vi "curve_fitter.vi"(8 "Path 4":path, 9 "Path 3":path, 10 "Path 2":path, 11 "Path":path) -> (0 "interleaved array":dbl[](array[numeric]), 1 "RMS":dbl, 2 "Standard Dev":dbl, 3 "Arithmetic Mean":dbl)   [LabVIEW 2019]
uses:
  <vilib>/Analysis/6fits.llb/Curve Fitting Criteria.ctl
  <vilib>/Utility/file.llb/Read Delimited Spreadsheet (string).vi
  <vilib>/Analysis/NI_AALPro.lvlib
panel:
  out "Total Samples":dbl
  out "Variance":dbl
  out "Array":dbl[][](array[numeric])
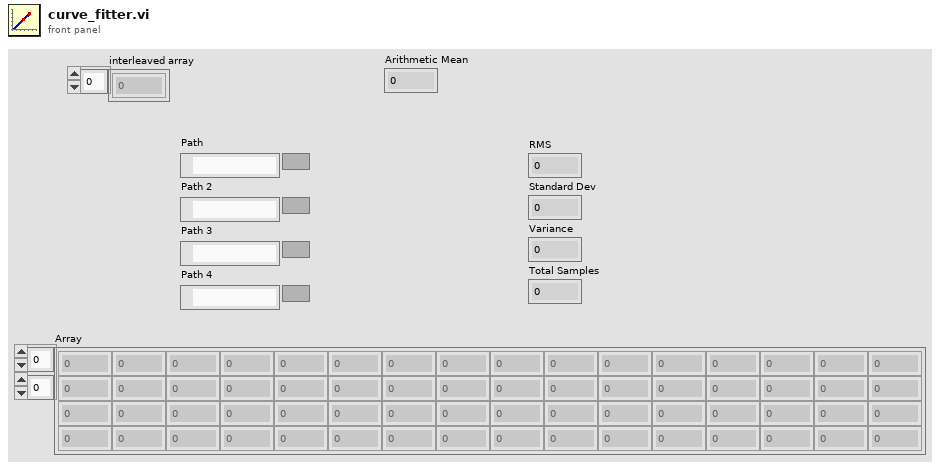
[diagram p1: front panel]
types:
  T1 = typedef "NI_AALPro.lvlib/Curve Fitting Criteria.ctl" = u16
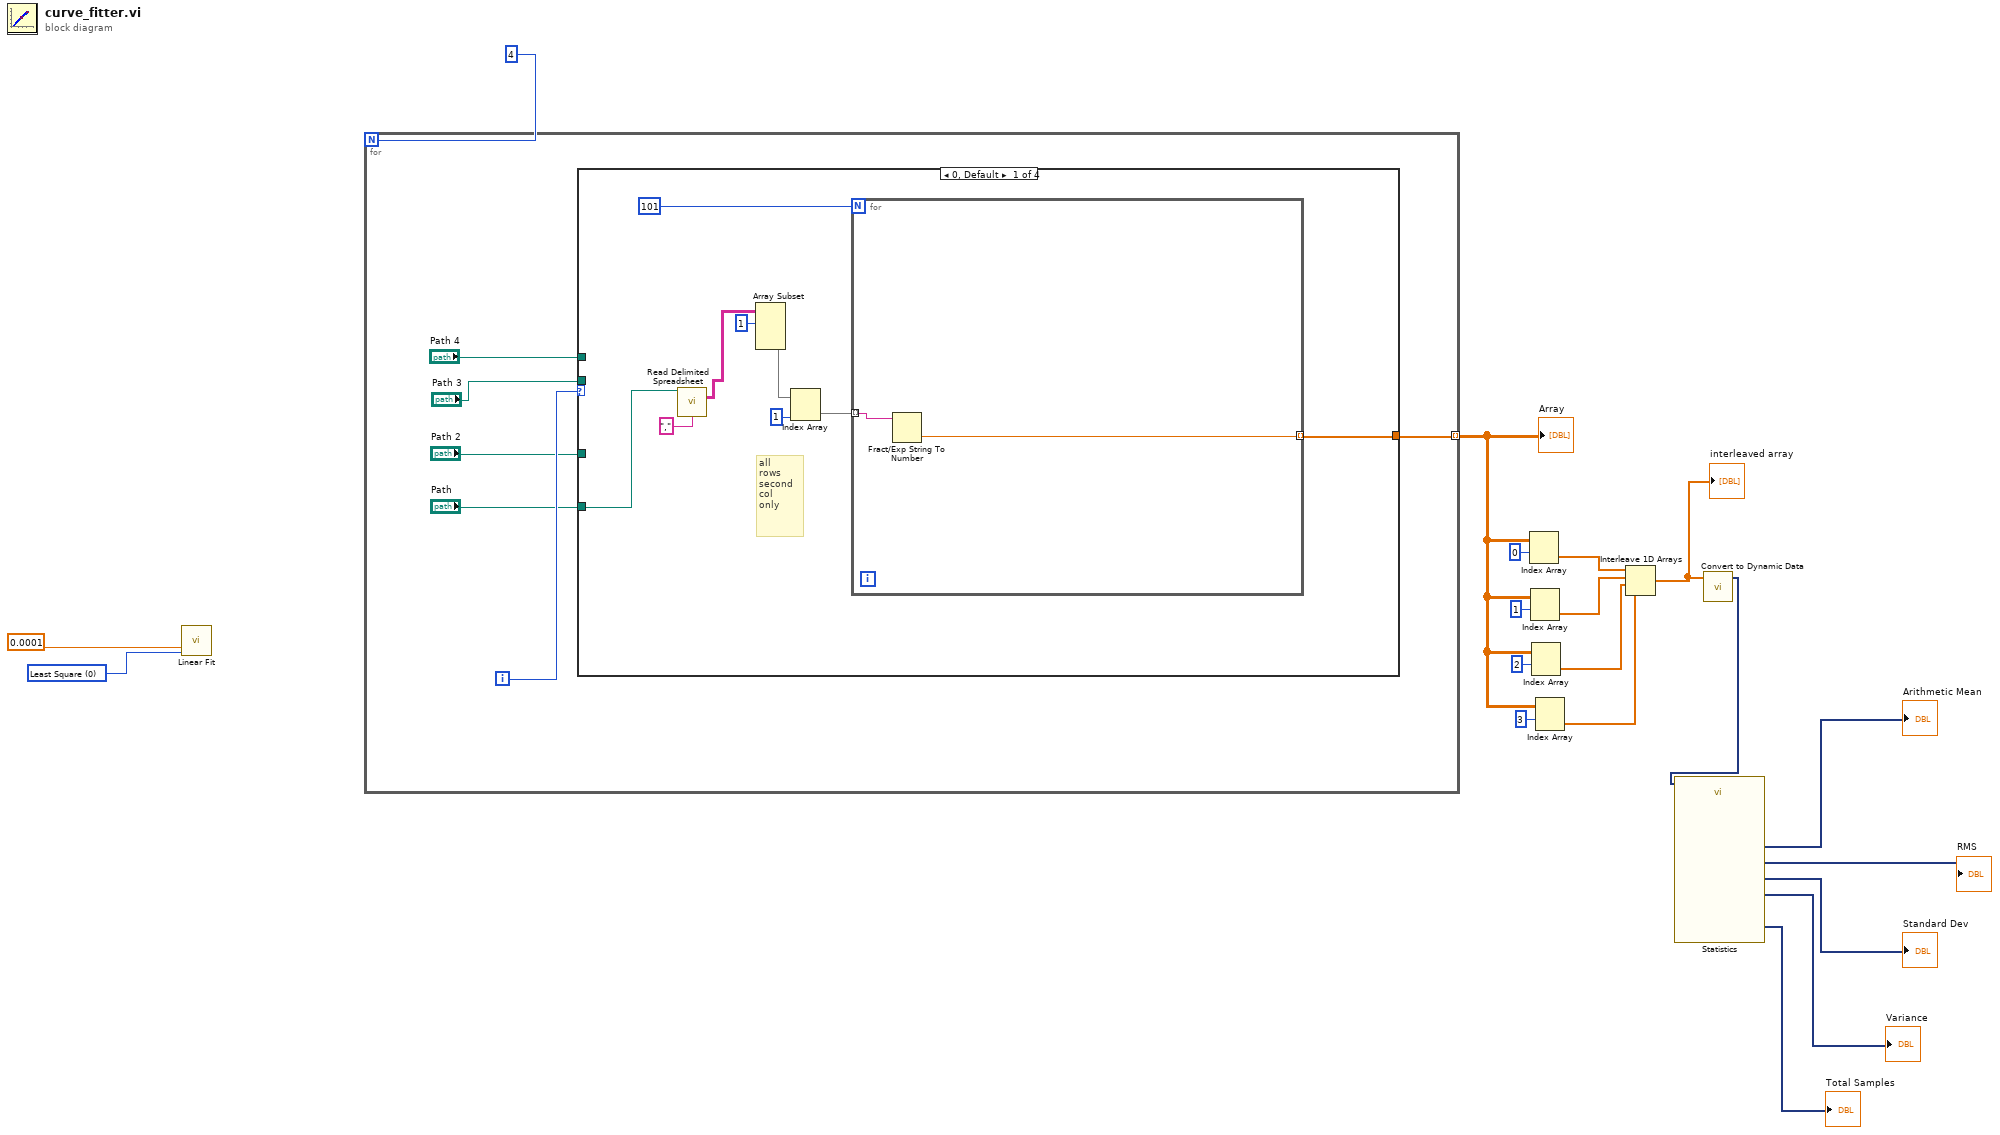
[diagram p0: block diagram]
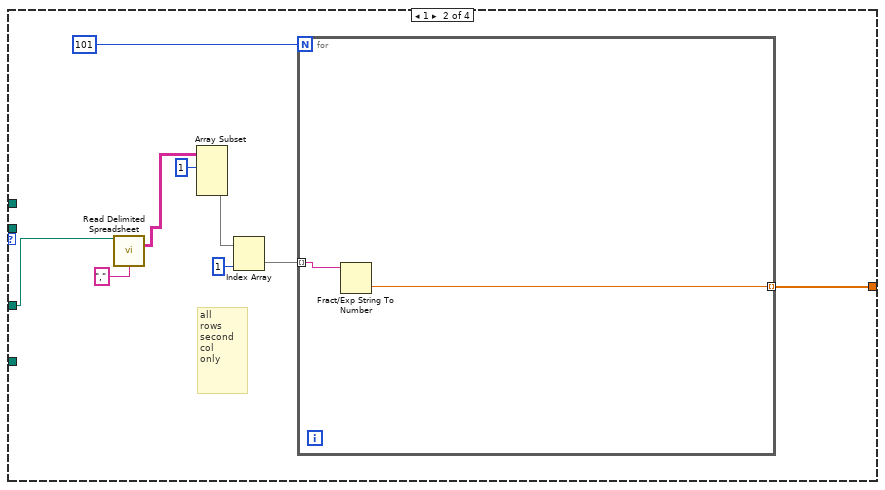
[diagram p2: hidden frame]
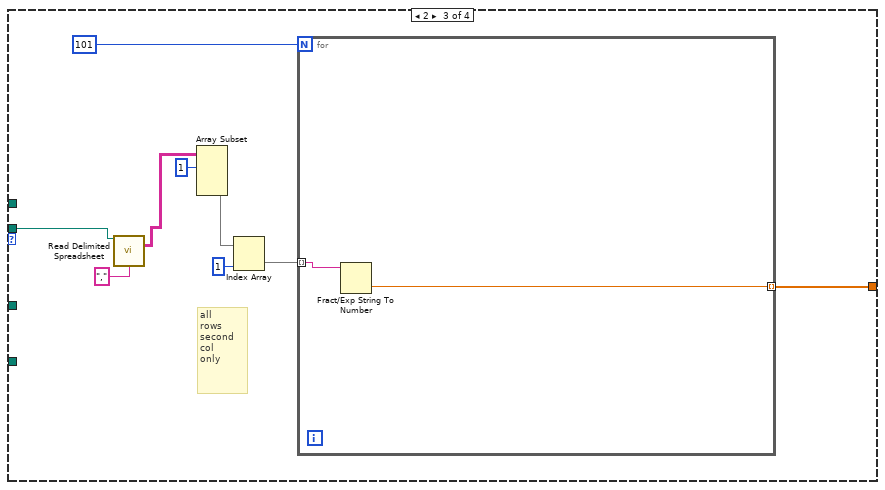
[diagram p3: hidden frame]
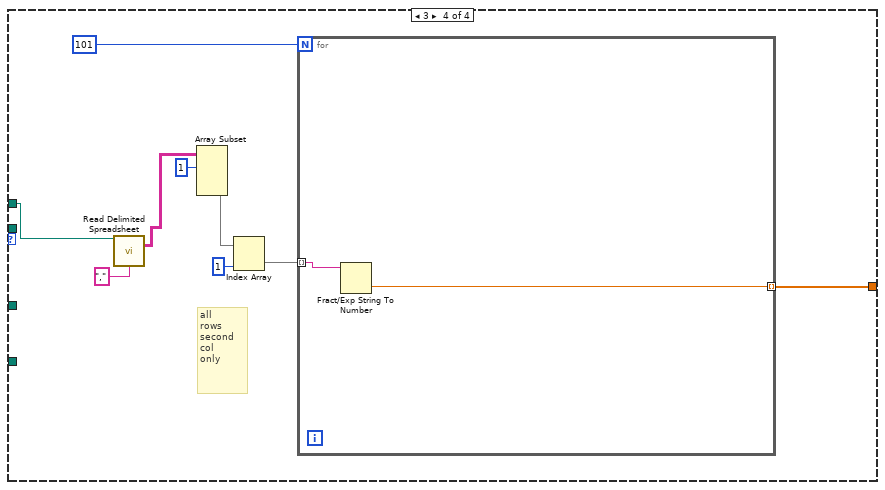
[diagram p4: hidden frame]
diagram:
  w19 = T1 0 items=["Least Square", "Least Absolute Residual", "Bisquare"] ("method")
  n1 = call <vilib>:"Linear Fit.vi"("tolerance"=0.0001, "method"=w19) -> ()  [unwired: 9 in, 5 out]
  n2 = for {
    N: 4 -> [_]
    tunnel: [w24] -> w13 mode=indexing
    i -> [w25]
    n3 = case shown="0, Default" w25 {
      tunnel: [w30 w41 w52 w63] -> w24
      tunnel: "Path 4" -> [_ _ _ w59]
      tunnel: "Path 3" -> [_ _ w48 _]
      tunnel: "Path 2" -> [_ w37 _ _]
      tunnel: "Path" -> [w26 _ _ _]
      frame 0, Default {
        # "all \nrows\nsecond \ncol\nonly"
        n4 = call-poly <vilib>:"Read Delimited Spreadsheet.vi"("file path (dialog if empty)"=w26, "delimiter (\\t)"="," ("delimiter (\\t)")) -> ("all rows"=w29:string[][])  [unwired: 8 in, 5 out]
        n5 = Array Subset(array=w29, index (row)=1 ("index")) -> (w27:string[][])  [unwired: 3 in]
        n6 = Index Array(array=w27, index (col)=1 ("disabled index (col)")) -> (element=w31:string[])  [unwired: 1 in]
        n7 = for {
          N: 101 -> [_]
          tunnel: w31 -> [w36] mode=indexing
          tunnel: [w35] -> w30 mode=indexing
          n8 = Fract/Exp String To Number(string=w36) -> (number=w35:dbl)  [unwired: 3 in, 1 out]
        }
      }
      frame 1 {
        # "all \nrows\nsecond \ncol\nonly"
        n9 = call-poly <vilib>:"Read Delimited Spreadsheet.vi"("file path (dialog if empty)"=w37, "delimiter (\\t)"="," ("delimiter (\\t)")) -> ("all rows"=w40:string[][])  [unwired: 8 in, 5 out]
        n10 = Array Subset(array=w40, index (row)=1 ("index")) -> (w38:string[][])  [unwired: 3 in]
        n11 = Index Array(array=w38, index (col)=1 ("disabled index (col)")) -> (element=w42:string[])  [unwired: 1 in]
        n12 = for {
          N: 101 -> [_]
          tunnel: w42 -> [w47] mode=indexing
          tunnel: [w46] -> w41 mode=indexing
          n13 = Fract/Exp String To Number(string=w47) -> (number=w46:dbl)  [unwired: 3 in, 1 out]
        }
      }
      frame 2 {
        # "all \nrows\nsecond \ncol\nonly"
        n14 = call-poly <vilib>:"Read Delimited Spreadsheet.vi"("file path (dialog if empty)"=w48, "delimiter (\\t)"="," ("delimiter (\\t)")) -> ("all rows"=w51:string[][])  [unwired: 8 in, 5 out]
        n15 = Array Subset(array=w51, index (row)=1 ("index")) -> (w49:string[][])  [unwired: 3 in]
        n16 = Index Array(array=w49, index (col)=1 ("disabled index (col)")) -> (element=w53:string[])  [unwired: 1 in]
        n17 = for {
          N: 101 -> [_]
          tunnel: w53 -> [w58] mode=indexing
          tunnel: [w57] -> w52 mode=indexing
          n18 = Fract/Exp String To Number(string=w58) -> (number=w57:dbl)  [unwired: 3 in, 1 out]
        }
      }
      frame 3 {
        # "all \nrows\nsecond \ncol\nonly"
        n19 = call-poly <vilib>:"Read Delimited Spreadsheet.vi"("file path (dialog if empty)"=w59, "delimiter (\\t)"="," ("delimiter (\\t)")) -> ("all rows"=w62:string[][])  [unwired: 8 in, 5 out]
        n20 = Array Subset(array=w62, index (row)=1 ("index")) -> (w60:string[][])  [unwired: 3 in]
        n21 = Index Array(array=w60, index (col)=1 ("disabled index (col)")) -> (element=w64:string[])  [unwired: 1 in]
        n22 = for {
          N: 101 -> [_]
          tunnel: w64 -> [w69] mode=indexing
          tunnel: [w68] -> w63 mode=indexing
          n23 = Fract/Exp String To Number(string=w69) -> (number=w68:dbl)  [unwired: 3 in, 1 out]
        }
      }
    }
  }
  "Array" <- w13
  n24 = Index Array(array=w13, index (row)=0) -> (element=w15:dbl[])  [unwired: 1 in]
  n25 = Index Array(array=w13, index (row)=1) -> (element=w14:dbl[])  [unwired: 1 in]
  n26 = Index Array(array=w13, index (row)=2) -> (element=w9:dbl[])  [unwired: 1 in]
  n27 = Index Array(array=w13, index (row)=3) -> (element=w8:dbl[])  [unwired: 1 in]
  n28 = Interleave 1D Arrays(w15, w14, w9, w8) -> (w7:dbl[])
  "interleaved array" <- w7
  n29 = call "Convert to Dynamic Data"("Array"=w7) -> ("Dynamic Data Type"=w6:dynamicdata)  [unwired: 3 in]
  n30 = call "Statistics"("Signals"=w6) -> ("Total Samples"=→"Total Samples":dynamicdata, "Variance"=→"Variance":dynamicdata, "Standard Dev"=→"Standard Dev":dynamicdata, "RMS"=→"RMS":dynamicdata, "Arithmetic Mean"=→"Arithmetic Mean":dynamicdata)  [unwired: 20 in, 2 out]
